vi "GetByManufacturer.vi"(8 "error in":errorcluster, 11 "ProductUnit in":refnum<class "ProductUnit.lvclass">) -> (0 "error out":errorcluster, 2 "ByManufacturer":string, 3 "ProductUnit out":refnum<class "ProductUnit.lvclass">)   [LabVIEW 2021, in "ProligentXMLGenerator.lvlib" / "ProductUnit.lvclass"]
doc: "Name of the original EMS provider or manufacturing site.\n\nThis attribute can't be updated after having been provided once.\n\nNon empty string restricted to 255 characters."
uses:
  ProductUnit.lvclass
  ProductUnit.lvclass/ProductUnit.ctl
  Base/NonEmptyString_255/NonEmptyString_255.lvclass
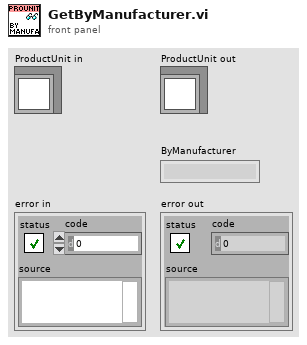
[diagram p1: front panel]
types:
  T1 = typedef "ProligentXMLGenerator.lvlib/ProductUnit.lvclass/Data.ctl" = cluster{"Name":string, "Characteristics":refnum<class "Characteristic.lvclass">[], "Documents":refnum<class "Document.lvclass">[], "CustomData":refnum<class "CustomData.lvclass">, "ProductUnitIdentifier":refnum<class "NonEmptyString_50.lvclass">, "ProductFullName":refnum<class "FullName.lvclass">, "Scrapped":refnum<class "Boolean.lvclass">, "ScrappedTime":refnum<class "DateTime.lvclass">, "CreationTime":refnum<class "DateTime.lvclass">, "ManufacturingTime":refnum<class "DateTime.lvclass">, "ByManufacturer":refnum<class "NonEmptyString_255.lvclass">, "TimeZoneInfoId":string}
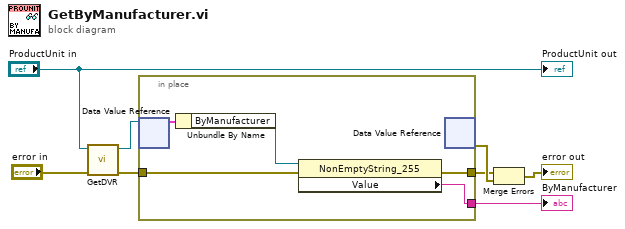
[diagram p0: block diagram]
diagram:
  n1 = call "GetDVR.vi"("error in"="error in", "ProductUnit in"="ProductUnit in") -> ("error out"=w2:errorcluster, "DVRReference"=w7:refnum<data-value>)  [unwired: 8 in]
  n2 = in-place "In Place Element Structure" {
    in-place-border: [w10] -> w6
    in-place-border: w2 -> [w11]
    in-place-border: [w9] -> w1
    n3 = in-place-dvr #1(w7) -> (w13:T1)  [unwired: 1 out]
    n4 = Unbundle By Name(w13) -> ("ByManufacturer"=w12:refnum<class "NonEmptyString_255.lvclass">)
    n5 = property on="Property Node" class="NonEmptyString_255"(reference=w12, error in=w11) -> (error out=w9:errorcluster, "Value"=w10:string)  [unwired: 1 out]
    n6 = in-place-dvr #1() -> (w8:errorcluster)  [unwired: 1 in, 1 out]
  }
  "ByManufacturer" <- w6
  n7 = Merge Errors(w1, w8) -> (→"error out":errorcluster)
  "ProductUnit out" <- "ProductUnit in"
